vi "Set Control.vi"(8 "error in (no error)":errorcluster, 9 "Output #":i32=1, 10 "Control":T1, 11 "Temperature Controller in":refnum<class "Temperature Controller.lvclass">) -> (0 "error out":errorcluster, 3 "Temperature Controller out":refnum<class "Temperature Controller.lvclass">)   [LabVIEW 2021, in "Temperature Controller.lvclass"]
uses:
  Temperature Controller.lvclass
  NHMFL_Core/Libraries/Instruments/Temperature Controller/Controls/Control Mode.ctl
  Read T ctl driver.vi
  Write T ctl driver.vi
  NHMFL_Core/Libraries/Instruments/Temperature Controller Driver/Temperature Controller Driver.lvclass
  Temperature Controller.lvclass/Temperature Controller.ctl
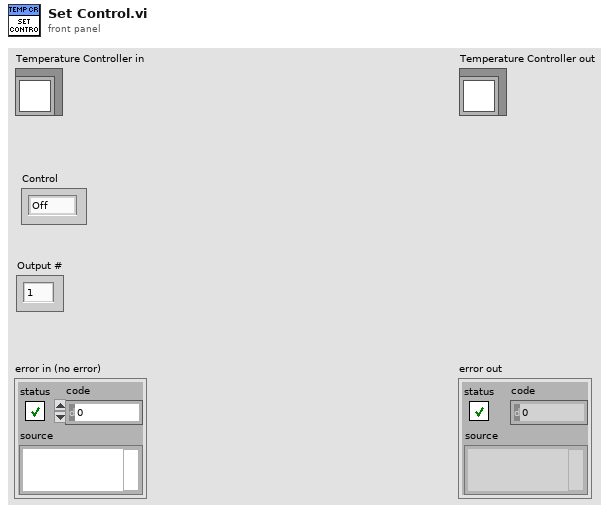
[diagram p1: front panel]
types:
  T1 = typedef "Control Mode.ctl" = enum16{"Off", "PID", "Ramp", "Manual", "Table"}
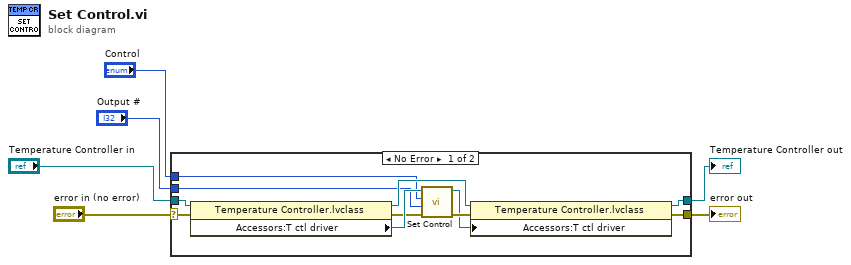
[diagram p0: block diagram]
diagram:
  n1 = case shown="No Error" "error in (no error)" {
    selector: "error in (no error)" -> [w9 w19]
    tunnel: [w8 w19] -> w5
    tunnel: [w12 w18] -> w3
    tunnel: "Temperature Controller in" -> [w11 w18]
    tunnel: "Control" -> [w10 _]
    tunnel: "Output #" -> [w7 _]
    frame No Error {
      n2 = property class="Temperature Controller.lvclass"(reference=w11, error in=w9) -> (reference out=w16:refnum<class "Temperature Controller.lvclass">, error out=w15:errorcluster, "Accessors:T ctl driver"=w17:refnum<class "Temperature Controller Driver.lvclass">)
      n3 = call-dynamic "Set Control.vi"("error in (no error)"=w15, "Output #"=w7, "Control"=w10, "Temperature Controller Driver in"=w17) -> ("error out"=w14:errorcluster, "Temperature Controller Driver out"=w13:refnum<class "Temperature Controller Driver.lvclass">)  [unwired: 6 in]
      n4 = property class="Temperature Controller.lvclass"(reference=w16, error in=w14, "Accessors:T ctl driver"=w13) -> (reference out=w12:refnum<class "Temperature Controller.lvclass">, error out=w8:errorcluster)
    }
    frame Error {
    }
  }
  "error out" <- w5
  "Temperature Controller out" <- w3
